vi "tcp.vi"() -> ()   [LabVIEW 2020]
uses:
  <vilib>/ErrorRing/Error Ring.xnode
panel:
  in  "Boolean":bool
  in  "stop":bool
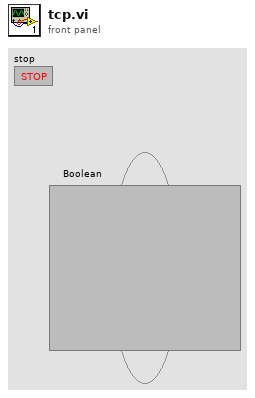
[diagram p1: front panel]
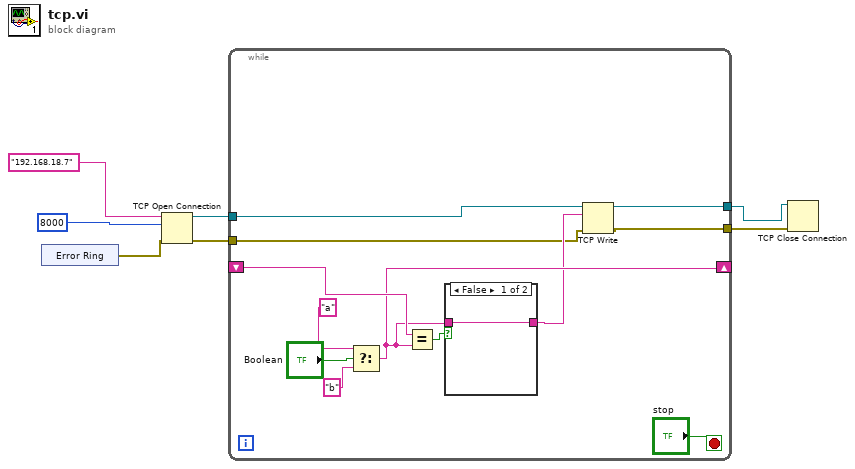
[diagram p0: block diagram]
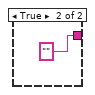
[diagram p2: hidden frame]
diagram:
  n1 = xnode "Error Ring"() -> ("error out"=w1:errorcluster)
  n2 = TCP Open Connection(address="192.168.18.7", remote port or service name=u16 8000, error in (no error)=w1) -> (connection ID=w7:refnum<k5>, error out=w6:errorcluster)  [unwired: 2 in]
  n3 = while {
    shift-right: [w13] -> _
    shift-left: _ -> [w14]
    tunnel: w7 -> [w11]
    tunnel: w6 -> [w10]
    tunnel: [w9] -> w5
    tunnel: [w8] -> w4
    stop <- "stop" stop-if-true
    n4 = Select(t="a", s="Boolean", f="b") -> (s? t:f=w13:string)
    n5 = Equal?(x=w14, y=w13) -> (x = y?=w15:bool)
    n6 = case shown="False" w15 {
      tunnel: [w20 ""] -> w12
      tunnel: w13 -> [w20 _]
      frame False {
      }
      frame True {
      }
    }
    n7 = TCP Write(connection ID=w11, data in=w12, error in (no error)=w10) -> (connection ID out=w9:refnum<k5>, error out=w8:errorcluster)  [unwired: 1 in, 1 out]
  }
  n8 = TCP Close Connection(connection ID=w5, error in (no error)=w4) -> ()  [unwired: 1 in, 2 out]
